vi "Power-measurement-Voltagedivider.vi"() -> ()   [LabVIEW 2018]
doc: "This example demonstrates how to continuously acquire buffered current measurements using a DAQmx device.\n\nFor instructions on how to connect your signals to the DAQ device, refer to your device documentation."
uses:
  <vilib>/Utility/error.llb/DialogType.ctl
  <vilib>/DAQmx/read.llb/DAQmx Read (Analog 1D Wfm NChan NSamp).vi
  <vilib>/DAQmx/create/channels.llb/DAQmx Create Channel (AI-Current-Basic).vi
  <vilib>/DAQmx/create/channels.llb/DAQmx Create Channel (AI-Voltage-Basic).vi
  <vilib>/DAQmx/configure/timing.llb/DAQmx Timing (Sample Clock).vi
  <vilib>/DAQmx/configure/task.llb/DAQmx Configure Logging (TDMS).vi
  <vilib>/DAQmx/miscellaneous.llb/DAQmx Fill In Error Info.vi
  <resource>/objmgr/daqmx.rc
panel:
  out "Waveform Voltage divider":waveform(dbl)(graph) caption="Voltage Divider"
  in  "Terminal Configuration 2":i32(ring)=-1 items=["default"=-1, "RSE"=10083, "NRSE"=10078, "Differential"=10106, "Pseudodifferential"=12529]
  in  "Max Voltage 2":dbl=5.0
  in  "Min Voltage 2":dbl=-5.0
  in  "Physical Channel 3":tag="Dev1/ai0"
  out "Waveform Current":waveform(dbl)(graph) caption="Shunt Currrent"
  out "Waveform GPIO Voltage":waveform(dbl)(graph) caption="GPIO Voltage"
  in  "Terminal Configuration":i32(ring)=-1 items=["default"=-1, "RSE"=10083, "NRSE"=10078, "Differential"=10106, "Pseudodifferential"=12529]
  in  "Max Voltage":dbl=5.0
  in  "Min Voltage":dbl=-5.0
  in  "Physical Channel 2":tag="Dev1/ai0"
  in  "Shunt Value (Ohms)":dbl=249.0 format="%0.2f"
  in  "Shunt Resistor":i32(ring)=-1 items=["default"=-1, "Internal"=10200, "External"=10167]
  in  "Stop":bool
  in  "TDMS File Path":path
  in  "Samples per Loop":i32=1000
  in  "Sample Rate":dbl=1000.0
  in  "Sample Clock Source":tag="OnboardClock"
  in  "Max Current (A)":dbl=0.02
  in  "Min Current (A)":dbl
  in  "Physical Channel":tag="Dev1/ai0"
  out "Actual Sample Rate":dbl=1000.0 format="%0.2f"
  in  "Logging Mode":i32(ring)=10231 items=["Off"=10231, "Log and Read"=15842]
  # "Acquired Data"
  # "GPIO Settings"
  # "Current Settings"
  # "Voltage Divider Settings"
  # "Timing Settings"
  # "Logging Settings"
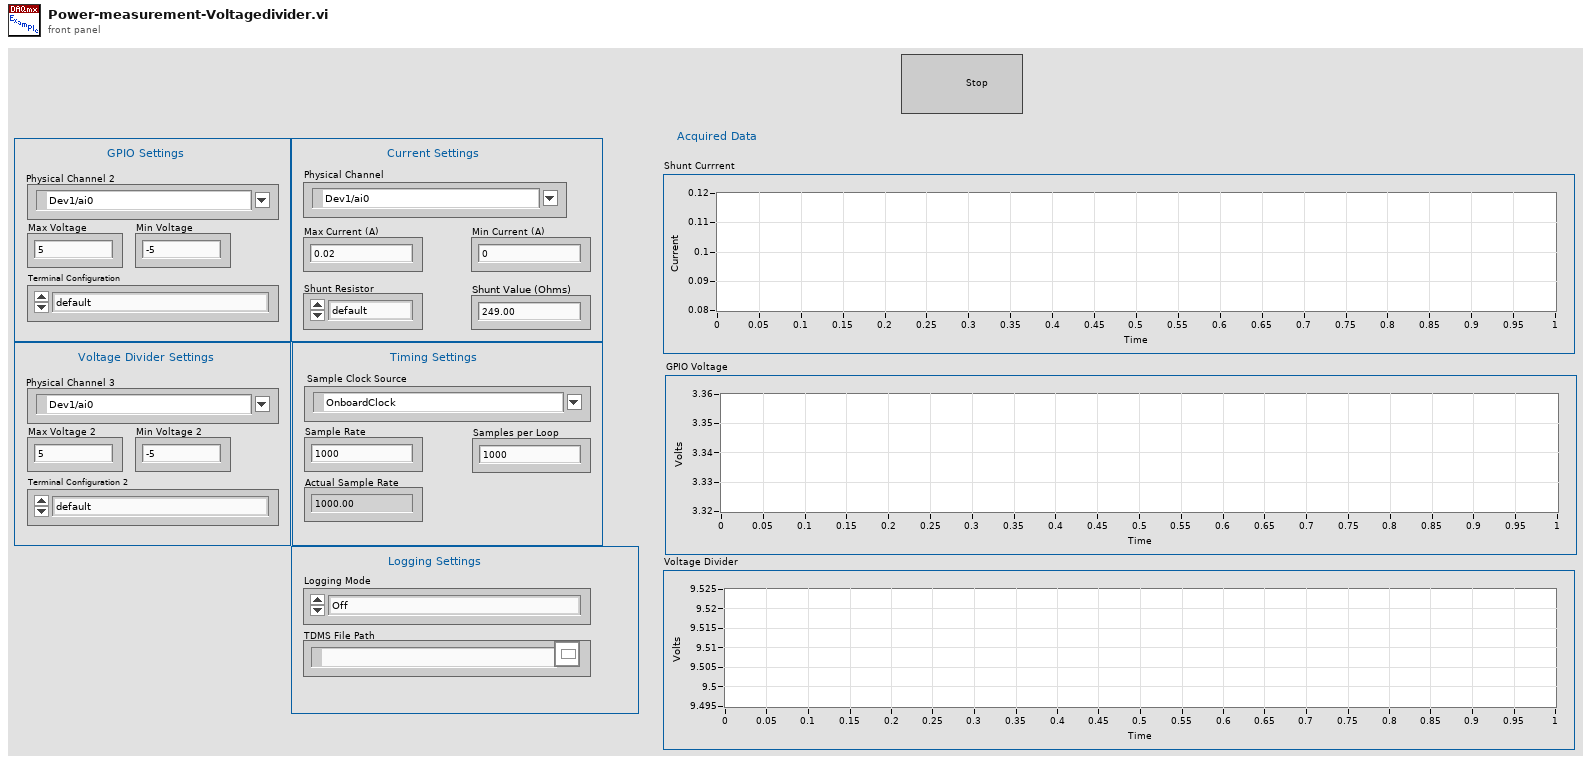
[diagram p1: front panel]
types:
  T1 = typedef "DialogType.ctl" = u16
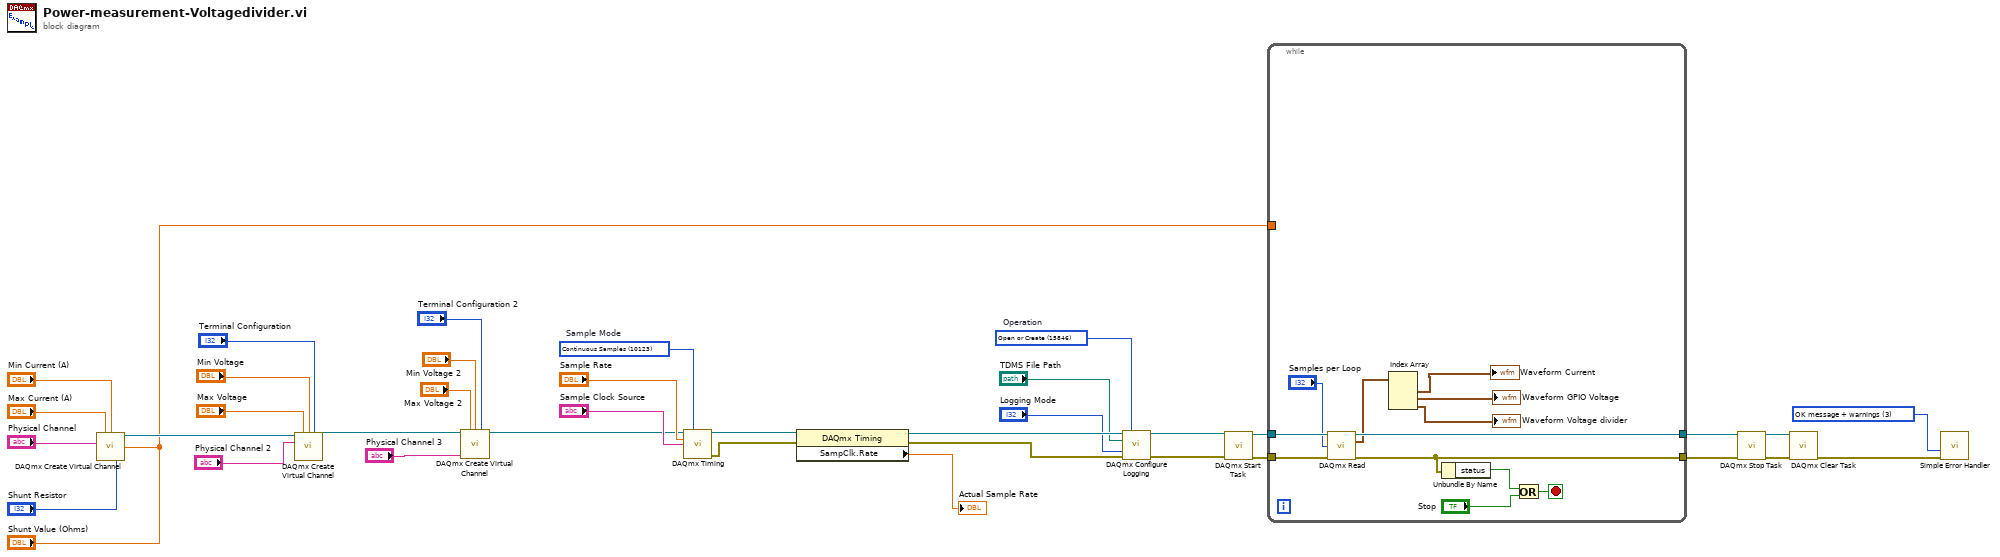
[diagram p0: block diagram]
diagram:
  w15 = T1 3 items=["no dialog", "OK message", "continue or stop message", "OK message + warnings", "continue/stop + warnings"] ("type of dialog (OK msg:1)")
  w32 = 15846 items=["Open"=10437, "Open or Create"=15846, "Create or Replace"=15847, "Create"=15848]  # Operation
  w35 = 10123 items=["Finite Samples"=10178, "Continuous Samples"=10123, "Hardware Timed Single Point"=12522]  # Sample Mode
  n1 = call-poly <vilib>:"DAQmx Create Virtual Channel.vi"("maximum value"="Max Current (A)", "minimum value"="Min Current (A)", "physical channels"="Physical Channel", "external shunt resistor value"="Shunt Value (Ohms)", "shunt resistor location"="Shunt Resistor") -> ("task out"=w8:refnum<k21>)  [unwired: 9 in, 1 out]
  n2 = call-poly <vilib>:"DAQmx Create Virtual Channel.vi"("task in"=w8, "maximum value"="Max Voltage", "minimum value"="Min Voltage", "input terminal configuration"="Terminal Configuration", "physical channels"="Physical Channel 2") -> ("task out"=w6:refnum<k21>)  [unwired: 9 in, 1 out]
  n3 = call-poly <vilib>:"DAQmx Create Virtual Channel.vi"("task in"=w6, "maximum value"="Max Voltage 2", "minimum value"="Min Voltage 2", "input terminal configuration"="Terminal Configuration 2", "physical channels"="Physical Channel 3") -> ("task out"=w5:refnum<k21>)  [unwired: 9 in, 1 out]
  n4 = call-poly <vilib>:"DAQmx Timing.vi"("task/channels in"=w5, "sample mode"=w35, "rate"="Sample Rate", "source"="Sample Clock Source") -> ("task out"=w37:refnum<k21>, "error out"=w36:errorcluster)  [unwired: 10 in]
  n5 = property class="DAQmx Timing"(reference=w37, error in=w36) -> (reference out=w34:refnum<k21>, error out=w33:errorcluster, "SampClk.Rate"=→"Actual Sample Rate":dbl)
  n6 = call-poly <vilib>:"DAQmx Configure Logging.vi"("task/channels in"=w34, "operation"=w32, "file path"="TDMS File Path", "logging mode"="Logging Mode", "error in"=w33) -> ("task out"=w14:refnum<k21>, "error out"=w13:errorcluster)  [unwired: 9 in]
  n7 = call <vilib>:"DAQmx Start Task.vi"("task/channels in"=w14, "error in"=w13) -> ("task out"=w31:refnum<k21>, "error out"=w30:errorcluster)  [unwired: 12 in]
  n8 = while {
    tunnel: w31 -> [w49]
    tunnel: w30 -> [w48]
    tunnel: [w45] -> w18
    tunnel: [w46] -> w19
    tunnel: "Shunt Value (Ohms)" -> [_]
    stop <- w47 stop-if-true
    n9 = call-poly <vilib>:"DAQmx Read.vi"("task/channels in"=w49, "number of samples per channel"="Samples per Loop", "error in"=w48) -> ("task out"=w46:refnum<k21>, "data"=w40:waveform(dbl)[], "error out"=w45:errorcluster)  [unwired: 10 in]
    n10 = Index Array(array=w40) -> (element #1=→"Waveform Current":waveform(dbl), element #2=→"Waveform GPIO Voltage":waveform(dbl), element #3=→"Waveform Voltage divider":waveform(dbl))  [unwired: 3 in]
    n11 = Unbundle By Name(w45) -> ("status"=w44:bool)
    n12 = Or(x=w44, y="Stop") -> (x .or. y?=w47:bool)
  }
  n13 = call <vilib>:"DAQmx Stop Task.vi"("task/channels in"=w19, "error in"=w18) -> ("task out"=w17:refnum<k21>, "error out"=w16:errorcluster)  [unwired: 12 in]
  n14 = call <vilib>:"DAQmx Clear Task.vi"("task in"=w17, "error in"=w16) -> ("error out"=w29:errorcluster)  [unwired: 13 in]
  n15 = call <vilib>:"Simple Error Handler.vi"("type of dialog (OK msg:1)"=w15, "error in (no error)"=w29) -> ()  [unwired: 3 in, 5 out]
